vi "UDP send.vi"(5 "port or service name":u16=37001, 7 "IP address":string="10.1.1.242", 8 "error in":errorcluster, 10 "Array":dbl[](array[numeric])=[0.0, 0.0, 0.0, 0.0, 0.0], 11 "connection ID in":refnum<k16>) -> (0 "error out":errorcluster, 3 "connection ID out":refnum<k16>, 6 "raw data":string)   [LabVIEW 2018]
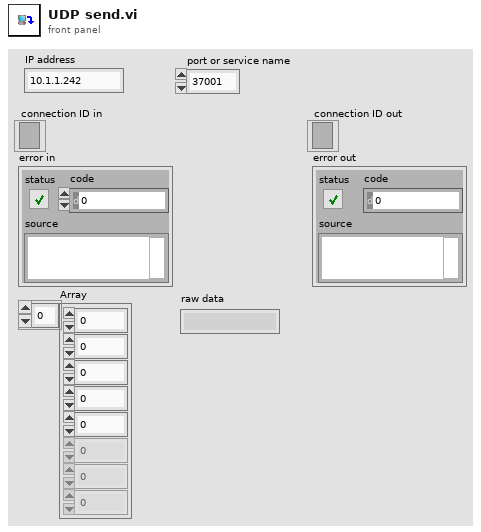
[diagram p1: front panel]
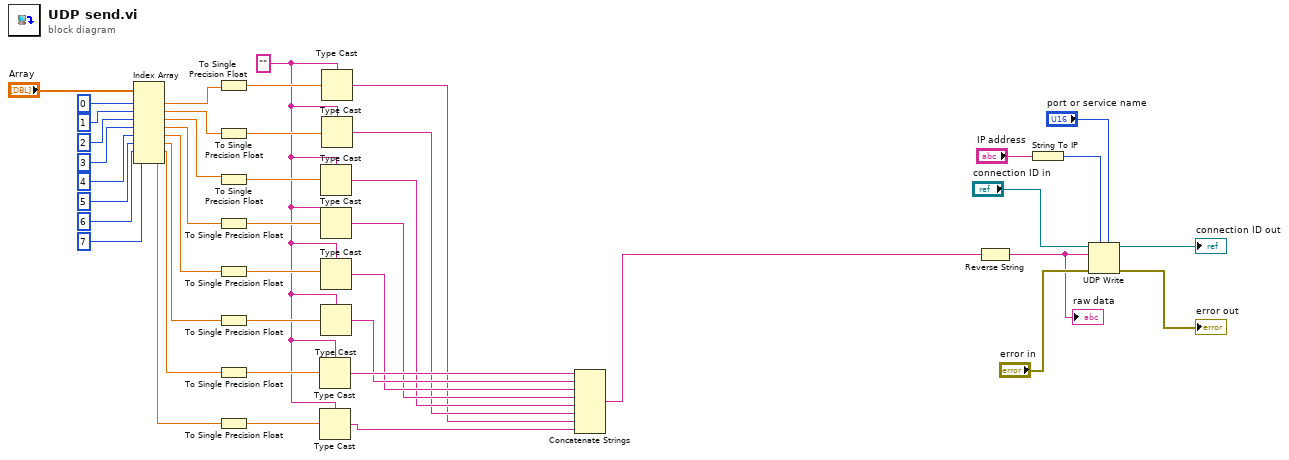
[diagram p0: block diagram]
diagram:
  w2 = "" ("reversed")
  n1 = Index Array(array="Array", index #1=0 ("index"), index #2=1 ("index"), index #3=2 ("index"), index #4=3 ("index"), index #5=4, index #6=5, index #7=6, index #8=7) -> (element #1=w31:dbl, element #2=w30:dbl, element #3=w29:dbl, element #4=w28:dbl, element #5=w19:dbl, element #6=w18:dbl, element #7=w17:dbl, element #8=w4:dbl)
  n2 = To Single Precision Float(number=w31) -> (single precision float=w39:sgl)
  n3 = To Single Precision Float(number=w30) -> (single precision float=w36:sgl)
  n4 = To Single Precision Float(number=w29) -> (single precision float=w37:sgl)
  n5 = To Single Precision Float(number=w28) -> (single precision float=w38:sgl)
  n6 = To Single Precision Float(number=w19) -> (single precision float=w16:sgl)
  n7 = To Single Precision Float(number=w18) -> (single precision float=w15:sgl)
  n8 = To Single Precision Float(number=w17) -> (single precision float=w14:sgl)
  n9 = To Single Precision Float(number=w4) -> (single precision float=w6:sgl)
  n10 = Type Cast(type=w2, x=w14) -> (*(type *) &x=w13:string)
  n11 = Type Cast(type=w2, x=w6) -> (*(type *) &x=w3:string)
  n12 = Type Cast(type=w2, x=w37) -> (*(type *) &x=w9:string)
  n13 = Type Cast(type=w2, x=w38) -> (*(type *) &x=w10:string)
  n14 = Type Cast(type=w2, x=w16) -> (*(type *) &x=w11:string)
  n15 = Type Cast(type=w2, x=w15) -> (*(type *) &x=w12:string)
  n16 = Type Cast(type=w2, x=w39) -> (*(type *) &x=w7:string)
  n17 = Type Cast(type=w2, x=w36) -> (*(type *) &x=w8:string)
  n18 = Concatenate Strings(w13, w12, w11, w10, w9, w8, w7, w3) -> (w43:string)
  n19 = Reverse String(1:w43) -> (0:w1:string)
  "raw data" <- w1
  n20 = String To IP(1:"IP address") -> (0:w42:u32)
  n21 = UDP Write(address=w42, port or service name="port or service name", connection ID="connection ID in", data in=w1, 8:"error in") -> (error out=→"error out":errorcluster, 3:→"connection ID out":refnum<k16>)  [unwired: 1 in]
